vi "Read From File.vi"(11 "file path (use dialog)":path) -> (3 "String":string)   [LabVIEW 2019]
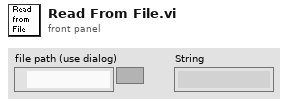
[diagram p1: front panel]
types:
  T1 = enum16{"open", "replace", "create", "open or create", "replace or create", "replace or create with confirmation"}
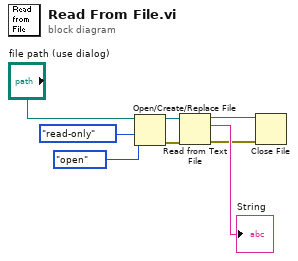
[diagram p0: block diagram]
diagram:
  n1 = Open/Create/Replace File(file path (use dialog)="file path (use dialog)", operation (0:open)=T1."open", access (0:read/write)=enum16{"read/write", "read-only", "write-only"}."read-only") -> (refnum out=w2:refnum<file>, error out=w1:errorcluster)  [unwired: 3 in, 1 out]
  n2 = Read from Text File(file (use dialog)=w2, error in=w1) -> (refnum out=w7:refnum<file>, text=→"String":string, error out=w6:errorcluster)  [unwired: 2 in, 1 out]
  n3 = Close File(refnum=w7, error in=w6) -> ()  [unwired: 2 out]
